vi "Post Actor Core Stop Sequencer Core.vi"(8 "error in (no error)":errorcluster, 11 "Sequencer Core in":refnum<class "Sequencer Core.lvclass">) -> (0 "error out":errorcluster, 3 "Sequencer Core out":refnum<class "Sequencer Core.lvclass">)   [LabVIEW 2020, in "Sequencer.lvlib" / "Sequencer Core.lvclass"]
uses:
  Sequencer Core.lvclass
  Sequencer Core.lvclass/Sequencer Core.ctl
  PPL/HDH.Actor Framework.Core.Actor.lvlibp/1abvi3w/vi.lib/ActorFramework/Stop Msg/Stop Msg.lvclass
  C:/Current projects/WS/PPL/HDH.Actor Framework.Core.Actor.lvlibp/1abvi3w/vi.lib/ActorFramework/Message/Message.lvclass
  PPL/HDH.Data.Generic.lvlibp/Data.lvclass
  Message Priority Queue/Message Priority Queue.lvclass
  PPL/HDH.Data.Generic.lvlibp/Synchronization/Notifier/Notifier.lvclass
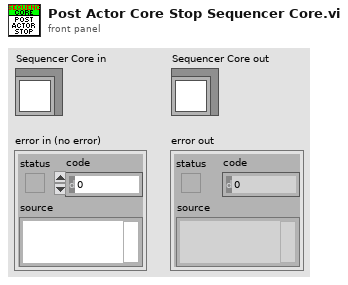
[diagram p1: front panel]
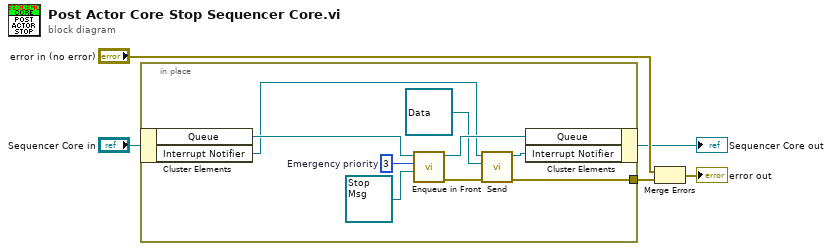
[diagram p0: block diagram]
diagram:
  n1 = in-place {
    in-place-border: [w7] -> w1
    w11 = 3  # Emergency priority
    n2 = in-place-cluster #1("Sequencer Core in") -> ("Queue"=w14:refnum<class "Message Priority Queue.lvclass">, "Interrupt Notifier"=w10:refnum<class "Notifier.lvclass">)
    n3 = call "Enqueue in Front.vi"("Message"=refnum<class "Stop Msg.lvclass"> refnum ("Actor Framework:Stop Msg"), "priority"=w11, "Priority Queue in"=w14) -> ("error out"=w8:errorcluster, "Priority Queue out"=w13:refnum<class "Message Priority Queue.lvclass">)  [unwired: 7 in]
    n4 = call "Send.vi"("error in (no error)"=w8, "Data Notification"=refnum<class "Data.lvclass"> refnum, "Notifier in"=w10) -> ("error out"=w7:errorcluster, "Notifier out"=w9:refnum<class "Notifier.lvclass">)  [unwired: 7 in]
    n5 = in-place-cluster #1("Queue"=w13, "Interrupt Notifier"=w9) -> (→"Sequencer Core out":refnum<class "Sequencer Core.lvclass">)
  }
  n6 = Merge Errors("error in (no error)", w1) -> (→"error out":errorcluster)
